vi "tcp_client_MW.vi"(0 "conn_id_in":refnum<k5>, 5 "addr":string="192.168.24.17", 7 "port":u16=10390, 11 "error in":errorcluster) -> (3 "status":bool, 4 "conn_id_out":refnum<k5>, 6 "Spill ID":i32, 8 "BOS Time":dbl format="%#.6f", 10 "EOS Time":dbl format="%#.6f", 15 "error out":errorcluster)   [LabVIEW 2019]
panel:
  out "Raw data array":string[](array[string])
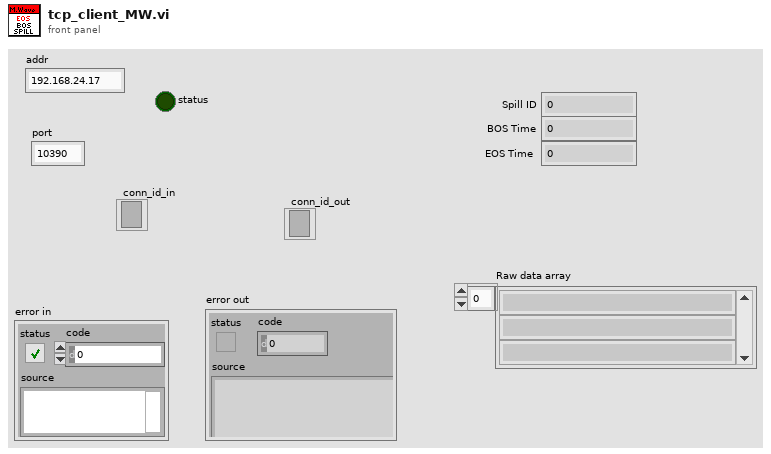
[diagram p1: front panel]
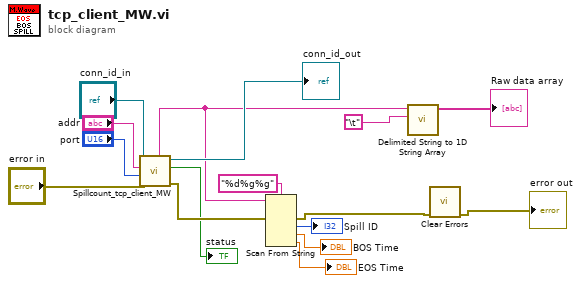
[diagram p0: block diagram]
diagram:
  n1 = call "Spillcount_tcp_client_MW.vi"("error in"="error in", "port"="port", "address"="addr", "conn_id_in"="conn_id_in") -> ("error out"=w14:errorcluster, "status"=→"status":bool, "conn_id_out"=→"conn_id_out":refnum<k5>, "data out"=w4:string)  [unwired: 3 in, 1 out]
  n2 = Scan From String(format string="%d%g%g", input string=w4, error in=w14) -> (error out=w2:errorcluster, output 1=→"Spill ID":i32, output 2=→"BOS Time":dbl, output 3=→"EOS Time":dbl)  [unwired: 4 in, 2 out]
  n3 = call <vilib>:"Delimited String to 1D String Array.vi"("delimiter"="\t", "delimited string"=w4) -> ("string array"=→"Raw data array":string[])  [unwired: 9 in]
  n4 = call <vilib>:"Clear Errors.vi"("error in (no error)"=w2) -> ("error out"=→"error out":errorcluster)  [unwired: 5 in, 1 out]
